vi "GetLibIconForVIIconOverlayFromVI.vi"(10 "Lib Refnum":refnum<vi>, 11 "VI Refnum":refnum<vi>) -> (1 "Owned by library?":bool, 3 "Library Icon For VI Overlay":T1)   [LabVIEW 2021]
uses:
  <vilib>/picture/picture.llb/imagedata.ctl
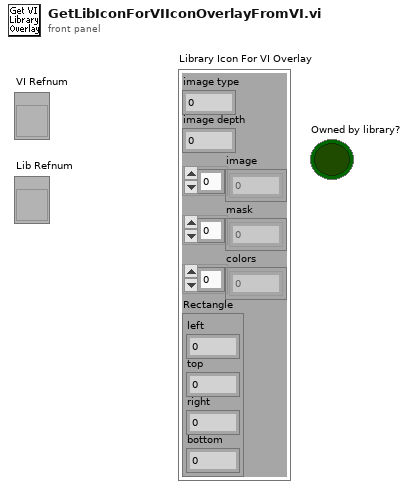
[diagram p1: front panel]
types:
  T1 = typedef "imagedata.ctl" = cluster{"image type":i32, "image depth":i32, "image":u8[], "mask":u8[], "colors":u32[], "Rectangle":cluster{"left":i16, "top":i16, "right":i16, "bottom":i16}}
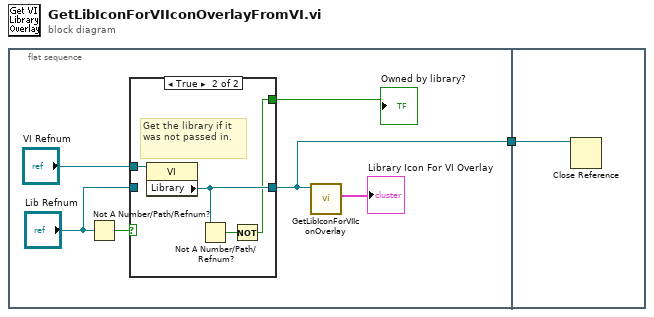
[diagram p0: block diagram]
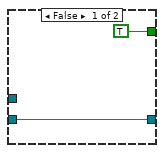
[diagram p2: hidden frame]
diagram:
  n1 = flat-sequence {
    tunnel: [w2] -> w1
    tunnel: w1 -> [w14]
    frame #0 {
      n2 = Not A Number/Path/Refnum?(number/path/refnum="Lib Refnum") -> (NaN/Path/Refnum?=w5:bool)
      n3 = case shown="True" w5 {
        tunnel: "VI Refnum" -> [_ w13]
        tunnel: [w9 w11] -> w2
        tunnel: "Lib Refnum" -> [w9 _]
        tunnel: [TRUE w10] -> w3
        frame False {
        }
        frame True {
          # "Get the library if it was not passed in."
          n4 = property class="VI"(reference=w13) -> ("Library"=w11:refnum<vi>)  [unwired: 1 in, 2 out]
          n5 = Not A Number/Path/Refnum?(number/path/refnum=w11) -> (NaN/Path/Refnum?=w12:bool)
          n6 = Not(x=w12) -> (.not. x?=w10:bool)
        }
      }
      "Owned by library?" <- w3
      n7 = call "GetLibIconForVIIconOverlay.vi"("Library"=w2) -> ("Library Icon For VI Overlay"=→"Library Icon For VI Overlay":T1)  [unwired: 10 out]
    }
    frame #1 {
      n8 = Close Reference(reference=w14) -> ()  [unwired: 1 in, 1 out]
    }
  }
